vi "SerialPort.Function_Query.vi"(5 "Timeout(ms)":i32=1000, 7 "Module Name":string="Serial Port", 8 "error in":errorcluster, 9 "EndStr":string="lhtx>", 10 "Cmd":string, 11 "Q In":refnum<queue>) -> (0 "error out":errorcluster, 2 "Data":string, 3 "Q Out":refnum<queue>)   [LabVIEW 2018]
uses:
  <vilib>/KATE/Queues/Q.Element.ctl
  Utils/Errors/Error.Error Code List.ctl
  <vilib>/KATE/Queues/Queue Utils.lvlib
panel:
  # "Serial Port Query"
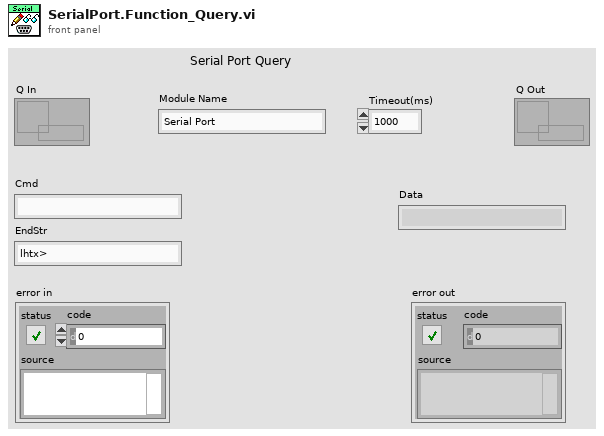
[diagram p1: front panel]
types:
  T1 = typedef "Error.Error Code List.ctl" = i32
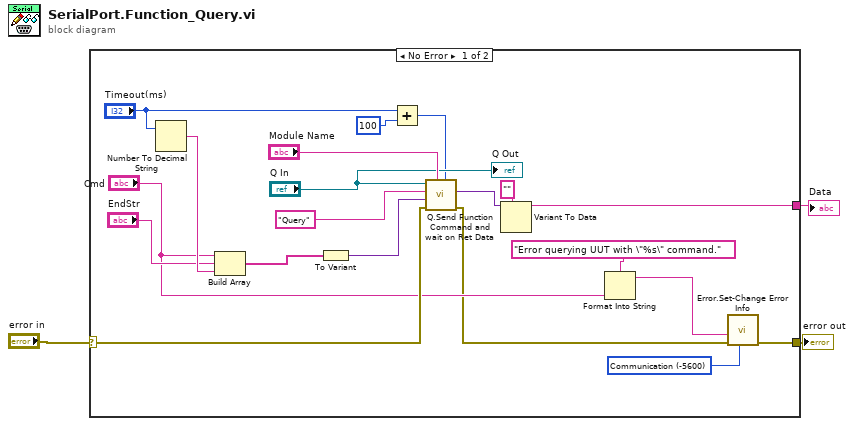
[diagram p0: block diagram]
diagram:
  n1 = case shown="No Error" "error in" {
    selector: "error in" -> [w21 w24]
    tunnel: [w5 w24] -> w2
    tunnel: [w10 _] -> w1
    frame No Error {
      w6 = T1 -5600 items=["No Error"=0, "Abort"=-2, "Misc"=-5000, "Fixture Error"=-5100, "File IO - General"=-5200, "FIle IO - Config Error"=-5201, "Instrument - General"=-5300, "Instrument - Serial Com"=-5301, "Instrument - Camera"=-5302, "Instrument - PS"=-5303, "Instrument - Oscilloscope"=-5304, "Instrument - Function Gen"=-5305, "Instrument - Load"=-5306, "Instrument - Meter"=-5307, "Instrument - Power Control"=-5308, "Instrument - Motion"=-5309, "Instrument - RF"=-5310, "System Exe"=-5400, "Image Processing"=-5500, "Communication"=-5600, "Script - Syntax Error"=-6000, "Script - Invalid Name or Param"=-6100, "Script - Timeout"=-6200, "Invalid Data"=-6300] ("Std Code")
      n2 = Number To Decimal String(number="Timeout(ms)") -> (decimal integer string=w15:string)  [unwired: 1 in]
      n3 = Build Array("Cmd", "EndStr", w15) -> (w13:string[])
      n4 = To Variant(anything=w13) -> (Variant=w20:variant)
      n5 = Add(x="Timeout(ms)", y=100) -> (x+y=w17:i32)
      n6 = call <vilib>:"Q.Send Function Command and wait on Ret Data.vi"("Timeout(ms)"=w17, "Q Name"="Module Name", "error in"=w21, "Data1"=w20, "Cmd"="Query", "Q In"="Q In") -> ("error out"=w4:errorcluster, "Ret"=w12:variant)  [unwired: 4 in]
      n7 = Variant To Data(type="", Variant=w12) -> (data=w10:string)  [unwired: 1 in, 1 out]
      n8 = Format Into String(format string="Error querying UUT with \"%s\" command.", "Cmd") -> (resulting string=w7:string)  [unwired: 2 in, 1 out]
      n9 = call "Error.Set-Change Error Info.vi"("Std Code"=w6, "error in"=w4, "Description"=w7) -> ("error out"=w5:errorcluster)  [unwired: 8 in]
      "Q Out" <- "Q In"
    }
    frame Error {
    }
  }
  "error out" <- w2
  "Data" <- w1
